vi "Read Source Path or URL.vi"(8 "error in (no error)":errorcluster, 11 "JSON Deserializer in":refnum<class "JSON Deserializer.lvclass">) -> (0 "error out":errorcluster, 2 "Source Path or URL":string, 3 "JSON Deserializer out":refnum<class "JSON Deserializer.lvclass">)   [LabVIEW 2020, in "JKI JSON Serialization.lvlib" / "JSON Deserializer.lvclass"]
uses:
  JSON Deserializer.lvclass
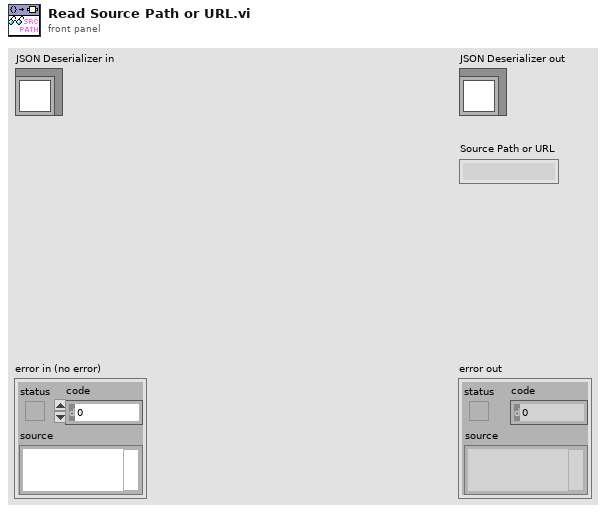
[diagram p1: front panel]
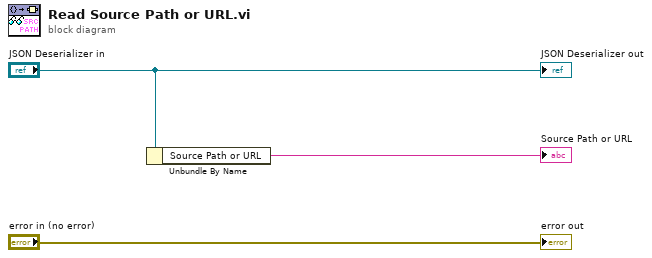
[diagram p0: block diagram]
diagram:
  n1 = Unbundle By Name("JSON Deserializer in") -> ("Source Path or URL"=→"Source Path or URL":string)
  "error out" <- "error in (no error)"
  "JSON Deserializer out" <- "JSON Deserializer in"
